vi "Read.vi"(8 "error in (no error)":errorcluster, 9 "timeout in ms (60 sec)":i32=60000, 11 "Result in":refnum<class "Task.lvclass">) -> (0 "error out":errorcluster, 1 "result error":errorcluster, 2 "Result value":variant, 3 "Result Out":refnum<class "Task.lvclass">, 4 "timed out?":bool)   [LabVIEW 2017, in "Futures.lvlib" / "Task.lvclass"]
doc: "Reads the value in the result.\n\nIf it has been resolved, then the result value will contain the result and the result error will be no error.\n\nIf it has been set to error, the Result value will be empty and the result error will contain the error that has been set."
uses:
  Task.lvclass
  Task.lvclass/Task.ctl
  <vilib>/ErrorRing/Error Ring.xnode
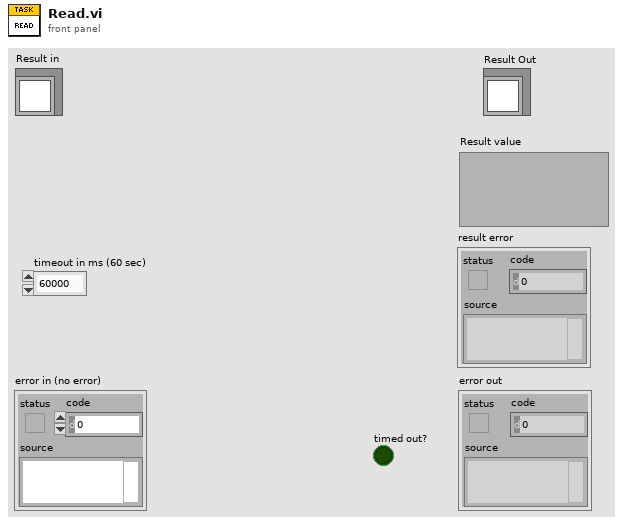
[diagram p1: front panel]
types:
  T1 = typedef "Futures.lvlib/Result.lvclass/Result Data.ctl" = cluster{"Type":T2, "Value":variant}
  T2 = typedef "Futures.lvlib/Result.lvclass/Result Type.ctl" = enum16{"Unresolved", "Ok", "Error"}
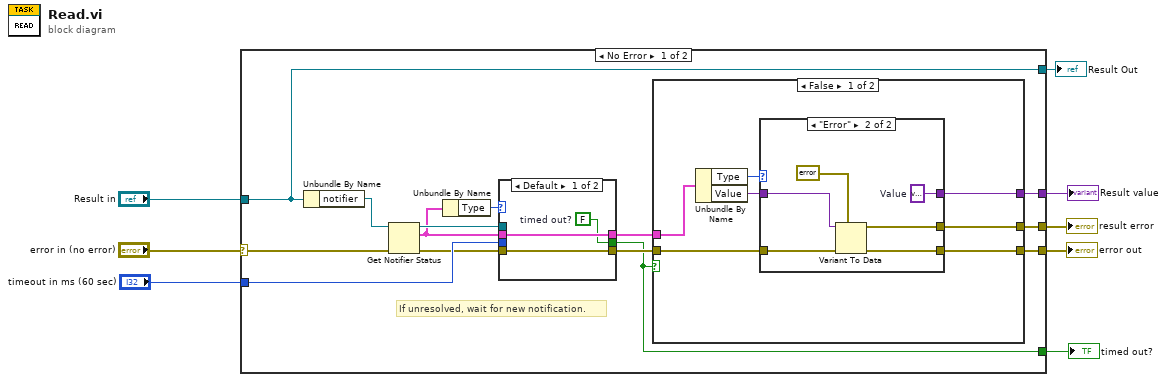
[diagram p0: block diagram]
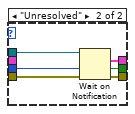
[diagram p2: hidden frame]
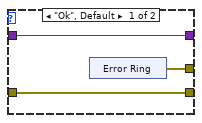
[diagram p3: hidden frame]
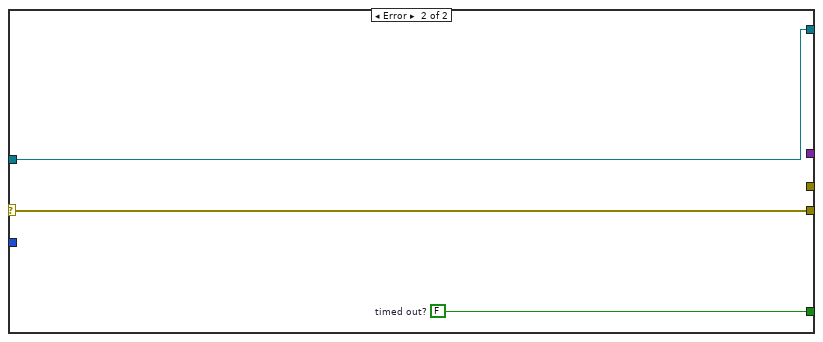
[diagram p5: hidden frame]
diagram:
  n1 = case shown="No Error" "error in (no error)" {
    selector: "error in (no error)" -> [w22 w52]
    tunnel: [w16 w52] -> w7
    tunnel: "Result in" -> [w14 w50]
    tunnel: "timeout in ms (60 sec)" -> [w21 _]
    tunnel: [w18 _] -> w4
    tunnel: [w17 _] -> w3
    tunnel: [w15 w51] -> w2
    tunnel: [w14 w50] -> w1
    frame No Error {
      # "If unresolved, wait for new notification."
      n2 = Unbundle By Name(w14) -> ("notifier"=w12:refnum<notifier>)
      n3 = Get Notifier Status(notifier=w12, error in (no error)=w22) -> (notifier out=w11:refnum<notifier>, current notification=w9:T1, error out=w13:errorcluster)  [unwired: 2 out]
      n4 = Unbundle By Name(w9) -> ("Type"=w10:T2)
      n5 = case shown="Default" w10 {
        tunnel: w21 -> [_ w31]
        tunnel: [w25 w30] -> w20
        tunnel: [w23 w29] -> w19
        tunnel: [w24 w28] -> w15
        tunnel: w13 -> [w23 w27]
        tunnel: w11 -> [_ w26]
        tunnel: w9 -> [w25 _]
        frame Default {
          w24 = FALSE  # timed out?
        }
        frame "Unresolved" {
          n6 = Wait on Notification(notifier=w26, timeout in ms (-1)=w31, error in (no error)=w27) -> (notification=w30:T1, timed out?=w28:bool, error out=w29:errorcluster)  [unwired: 1 in, 1 out]
        }
      }
      n7 = case shown="False" w15 {
        tunnel: w20 -> [w38 _]
        tunnel: w19 -> [w35 w49]
        tunnel: [w33 _] -> w18
        tunnel: [w32 _] -> w17
        tunnel: [w34 w49] -> w16
        frame False {
          n8 = Unbundle By Name(w38) -> ("Type"=w37:T2, "Value"=w36:variant)
          n9 = case shown="\"Error\"" w37 {
            tunnel: w36 -> [w41 w46]
            tunnel: w35 -> [w40 w48]
            tunnel: [w40 w47] -> w34
            tunnel: [w39 w44] -> w33
            tunnel: [w41 w43] -> w32
            frame "Ok", Default {
              n10 = xnode "Error Ring"() -> ("error out"=w39:errorcluster)
            }
            frame "Error" {
              w43 = variant  # Value
              n11 = Variant To Data(error in=w48, type=errorcluster {"status"=FALSE, "code"=0, "source"=""} ("error in (no error)"), Variant=w46) -> (data=w44:errorcluster, error out=w47:errorcluster)
            }
          }
        }
        frame True {
        }
      }
    }
    frame Error {
      w51 = FALSE  # timed out?
    }
  }
  "error out" <- w7
  "Result value" <- w3
  "result error" <- w4
  "timed out?" <- w2
  "Result Out" <- w1
